vi "FTW-ActorConfig-FormatActorVIName.vi"(0 "FTW Config String In":string="{}", 7 "Actor VI Name":string, 11 "error in":errorcluster) -> (4 "FTW Config String":string, 15 "error out":errorcluster)   [LabVIEW 2015]
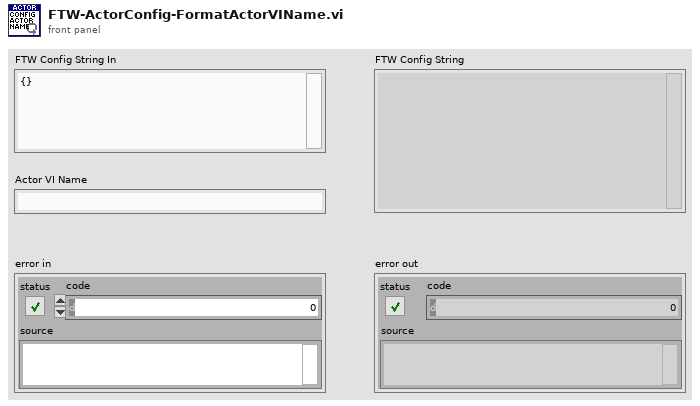
[diagram p1: front panel]
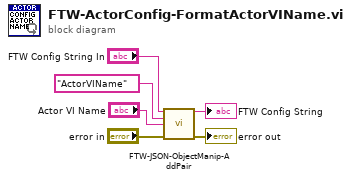
[diagram p0: block diagram]
diagram:
  n1 = call "FTW-JSON-ObjectManip-AddPair.vi"("Input JSON Object"="FTW Config String In", "Key"="ActorVIName", "Value"="Actor VI Name", "error in"="error in") -> ("Output JSON Object"=→"FTW Config String":string, "error out"=→"error out":errorcluster)  [unwired: 10 in]
